vi "Insert Children.vi"(6 "Label Names":string[](array[string]), 7 "OpenMetrics Compliant?":bool=TRUE, 8 "error in (no error)":errorcluster, 10 "Metric Name":string, 11 "Histogram in":refnum<class "Histogram.lvclass">) -> (0 "error out":errorcluster, 3 "Histogram out":refnum<class "Histogram.lvclass">)   [LabVIEW 2020, in "Metrics.lvlib" / "Histogram.lvclass"]
uses:
  Histogram.lvclass
  gauge/Gauge.lvclass
  C:/Github-locals/PromVIEW/src/metrics/metric/Metric.lvclass
  metric/Metric.lvclass/Metric.ctl
  Histogram.lvclass/Histogram.ctl
  metric/Write Name.vi
  metric/Write Label Names.vi
  metric/Validate Name.vi
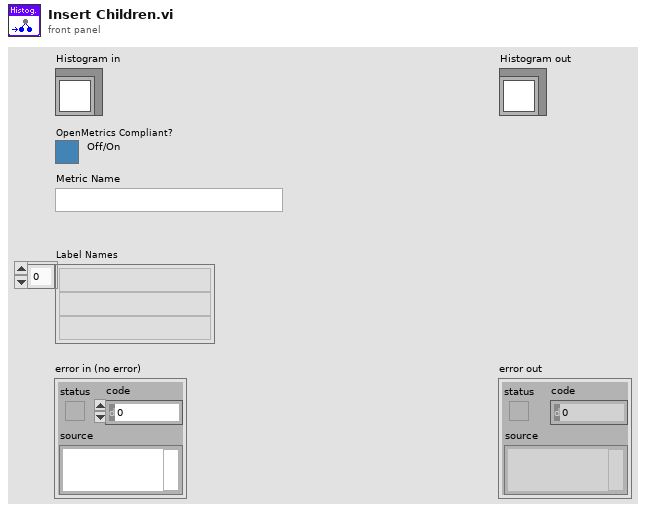
[diagram p1: front panel]
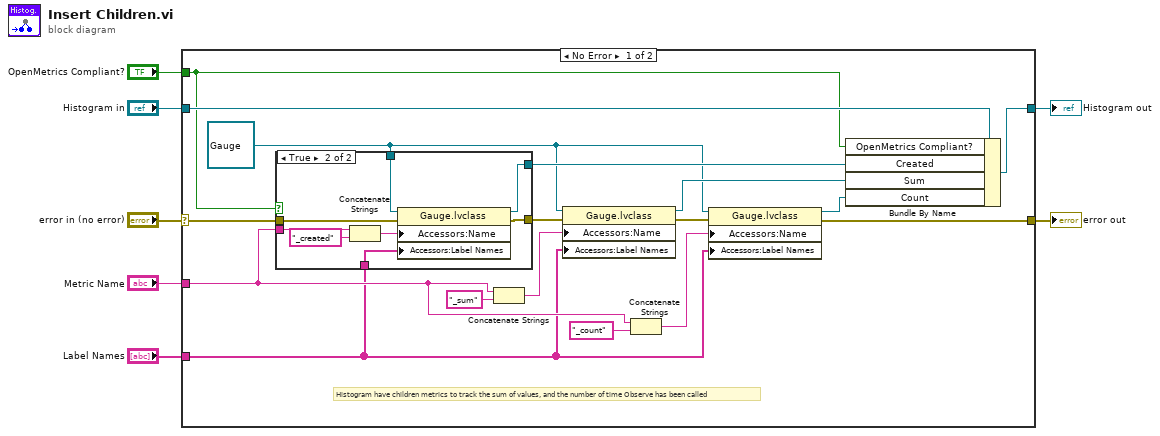
[diagram p0: block diagram]
diagram:
  n1 = case shown="No Error" "error in (no error)" {
    selector: "error in (no error)" -> [w10 w35]
    tunnel: [w9 w35] -> w6
    tunnel: [w23 w34] -> w4
    tunnel: "Histogram in" -> [w24 w34]
    tunnel: "Metric Name" -> [w19 _]
    tunnel: "Label Names" -> [w15 _]
    tunnel: "OpenMetrics Compliant?" -> [w8 _]
    frame No Error {
      w11 = refnum<class "Gauge.lvclass"> refnum ("Metrics.lvlib:Gauge.lvclass")
      # "Histogram have children metrics to track the sum of values, and the number of time Observe has been called"
      n2 = case shown="True" w8 {
        tunnel: w19 -> [_ w31]
        tunnel: [w25 w30] -> w18
        tunnel: w15 -> [_ w29]
        tunnel: [_ w28] -> w14
        tunnel: w11 -> [_ w27]
        tunnel: w10 -> [w25 w26]
        frame False {
        }
        frame True {
          n3 = Concatenate Strings(w31, "_created" ("string")) -> (w32:string)
          n4 = property class="Gauge.lvclass"(reference=w27, error in=w26, "Accessors:Name"=w32, "Accessors:Label Names"=w29) -> (reference out=w28:refnum<class "Gauge.lvclass">, error out=w30:errorcluster)
        }
      }
      n5 = Concatenate Strings(w19, "_sum" ("string")) -> (w20:string)
      n6 = property class="Gauge.lvclass"(reference=w11, error in=w18, "Accessors:Name"=w20, "Accessors:Label Names"=w15) -> (reference out=w13:refnum<class "Gauge.lvclass">, error out=w17:errorcluster)
      n7 = Concatenate Strings(w19, "_count" ("string")) -> (w16:string)
      n8 = property class="Gauge.lvclass"(reference=w11, error in=w17, "Accessors:Name"=w16, "Accessors:Label Names"=w15) -> (reference out=w12:refnum<class "Gauge.lvclass">, error out=w9:errorcluster)
      n9 = Bundle By Name(cluster=w24, "OpenMetrics Compliant?"=w8, "Created"=w14, "Sum"=w13, "Count"=w12) -> (w23:refnum<class "Histogram.lvclass">)
    }
    frame Error {
    }
  }
  "error out" <- w6
  "Histogram out" <- w4
